vi "Get Identifier.vi"(8 "error in":errorcluster, 11 "Ballard ARINC-429 Execution Unit in":refnum<class "Ballard ARINC-429 Execution Unit.lvclass">) -> (0 "error out":errorcluster, 2 "identifier":string, 3 "Ballard ARINC-429 Execution Unit out":refnum<class "Ballard ARINC-429 Execution Unit.lvclass">)   [LabVIEW 2020, in "Communication Bus Template Engine.lvlib" / "Implementation.lvlib" / "Ballard ARINC-429 Execution Unit.lvclass"]
uses:
  Ballard ARINC-429 Execution Unit.lvclass
  Ballard ARINC-429 Execution Unit.lvclass/Ballard ARINC-429 Execution Unit.ctl
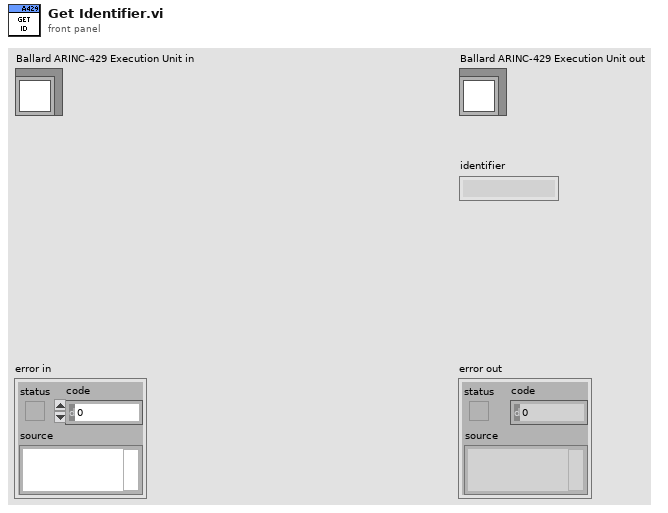
[diagram p1: front panel]
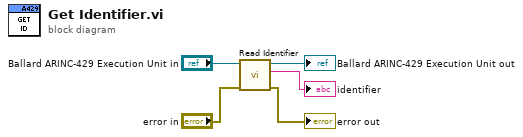
[diagram p0: block diagram]
diagram:
  n1 = call "Read Identifier.vi"("error in"="error in", "Ballard ARINC-429 Execution Unit in"="Ballard ARINC-429 Execution Unit in") -> ("error out"=→"error out":errorcluster, "identifier"=→"identifier":string, "Ballard ARINC-429 Execution Unit out"=→"Ballard ARINC-429 Execution Unit out":refnum<class "Ballard ARINC-429 Execution Unit.lvclass">)  [unwired: 7 in]
